vi "Teleop.vi"(10 "Match Info":T1={"Autonomous Elapsed Seconds"=0.0, "TeleOp Elapsed Seconds"=0.0, "Disabled Elapsed Seconds"=0.0, "Visited Autonomous"=FALSE, "Visited TeleOp"=FALSE, "Visited Disabled"=FALSE, "Autonomous Settings"={"Autonomous Style"=enum."Independent", "VI Refnum"=refnum}}, 11 "Call Context":T2) -> ()   [LabVIEW 2012]
doc: "This VI is called for each TeleOp packet received from the DS where the robot is not disabled. It is often used to read from the joysticks and update I/O or to update setpoints for timed control loops. It should complete and return within 20 milliseconds or it may miss DS packets."
uses:
  <vilib>/Rock Robotics/WPI/DriverStation/WPI_DriverStationDerivedRobotMode.ctl
  <vilib>/Rock Robotics/WPI/DriverStation/WPI_DriverStationMatch Info.ctl
  <vilib>/Rock Robotics/WPI/Relay/WPI_RelayValue.ctl
  Robot Global Data.vi
  <vilib>/Rock Robotics/WPI/Joystick/WPI_JoystickGetSetRefNum.vi
panel:
  in  "Hold":dbl=85.0
  in  "Allow Latch":dbl=25.0
  in  "Ext Const":dbl=0.5
  in  "Dep Const":dbl=0.5
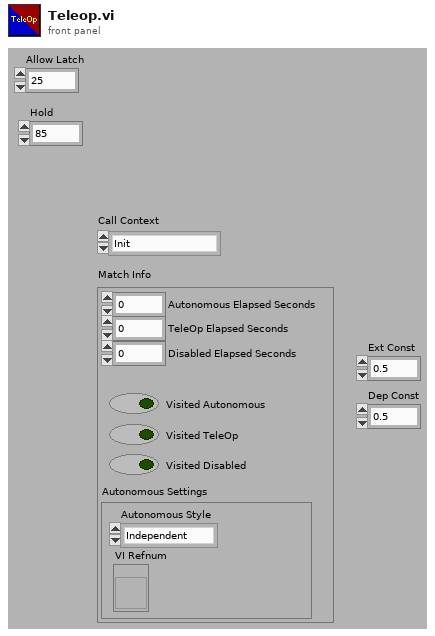
[diagram p1: front panel]
types:
  T1 = typedef "WPI_DriverStationMatch Info.ctl" = cluster{"Autonomous Elapsed Seconds":dbl, "TeleOp Elapsed Seconds":dbl, "Disabled Elapsed Seconds":dbl, "Visited Autonomous":bool, "Visited TeleOp":bool, "Visited Disabled":bool, "Autonomous Settings":cluster{"Autonomous Style":enum16{"Iterative", "Independent"}, "VI Refnum":refnum<vi>}}
  T2 = typedef "WPI_DriverStationDerivedRobotMode.ctl" = enum16{"Init", "Execute", "Stop"}
  T3 = typedef "WPI_RelayValue.ctl" = enum16{"Off", "On", "Forward", "Reverse"}
  T4 = typedef "WPI_ServoDeviceRef.ctl" = cluster{"DeviceStatus":errorcluster, "Digital Module":T5, "PWM Channel":T6, "DeadBand":T7}
  T5 = typedef "FPGA_TypedefDigitalModule.ctl" = enum16{"Digital Module 1", "Digital Module 2"}
  T6 = typedef "FPGA_DIOPWMChannel.ctl" = enum8{"PWM 1", "PWM 2", "PWM 3", "PWM 4", "PWM 5", "PWM 6", "PWM 7", "PWM 8", "PWM 9", "PWM 10", "Invalid"}
  T7 = typedef "WPI_PWMDeadband.ctl" = cluster{"Name":string, "maxPositivePwm":i32, "minPositivePwm":i32, "centerPwm":i32, "maxNegativePwm":i32, "minNegativePwm":i32, "angularRange":u16}
  T8 = typedef "WPI_MotorControlDeviceRef.ctl" = cluster{"DeviceStatus":errorcluster, "Type":enum16{"PWM", "CAN"}, "PWM":cluster{"Digital Module":T5, "PWM Channel":T6, "DeadBand":T7}, "CAN":cluster{"Device Number":u8, "Control Mode":T9, "Semaphore":T10, "Max Vout":dbl}, "Invert":bool, "TransformRef":T11, "InvTransformRef":T11}
  T9 = typedef "WPI_CANJaguar_ControlMode.ctl" = enum8{"Percent VBus", "Current", "Speed", "Position", "Voltage"}
  T10 = typedef "Semaphore RefNum" = refnum<k1>
  T11 = typedef "WPI_PWMTransform_ConPane.ctl" = refnum<vi>
  T12 = cluster{"Driver Station Digital Input (1-8)[0]":bool, "Driver Station Digital Input (1-8)[1]":bool, "Driver Station Digital Input (1-8)[2]":bool, "Driver Station Digital Input (1-8)[3]":bool, "Driver Station Digital Input (1-8)[4]":bool, "Driver Station Digital Input (1-8)[5]":bool, "Driver Station Digital Input (1-8)[6]":bool, "Driver Station Digital Input (1-8)[7]":bool, "Driver Station Digital Input (1-8)[8]":bool}
  T13 = cluster{"Right Servo High":dbl, "Right Servo Mid":dbl, "Right Servo Low":dbl, "Left Servo High":dbl, "Left Servo Mid":dbl, "Left Servo Low":dbl}
  T14 = typedef "WPI_DigitalInputDevRef.ctl" = cluster{"DevStatus":errorcluster, "DIO Channel":T15, "Digital Module":T5}
  T15 = typedef "FPGA_DIOChannel.ctl" = enum8{"DIO 1", "DIO 2", "DIO 3", "DIO 4", "DIO 5", "DIO 6", "DIO 7", "DIO 8", "DIO 9", "DIO 10", "DIO 11", "DIO 12", "DIO 13", "DIO 14", "Invalid"}
  T16 = typedef "WPI_JoystickDevRef.ctl" = cluster{"Device":T17}
  T17 = typedef "WPI_JoystickDeviceEnum.ctl" = enum16{"USB 1", "USB 2", "USB 3", "USB 4", "Kinect 1", "Kinect 2"}
  T18 = cluster{"axis 1 (x)":dbl, "axis 2 (y)":dbl, "axis 3 (throttle)":dbl, "axis 4":dbl, "axis 5":dbl, "axis 6":dbl}
  T19 = typedef "WPI_JoystickButtonState.ctl" = cluster{"Button 1":bool, "Button 2":bool, "Button 3":bool, "Button 4":bool, "Button 5":bool, "Button 6":bool, "Button 7":bool, "Button 8":bool, "Button 9":bool, "Button 10":bool, "Button 11":bool, "Button 12":bool}
  T20 = typedef "WPI_RelayDevRef.ctl" = cluster{"DevStatus":errorcluster, "Relay Channel":T21, "Digital Module":T5, "Relay Direction":T22}
  T21 = typedef "FPGA_DIORelayChannel.ctl" = enum8{"Relay 1", "Relay 2", "Relay 3", "Relay 4", "Relay 5", "Relay 6", "Relay 7", "Relay 8", "Invalid"}
  T22 = typedef "WPI_RelayDirection.ctl" = enum16{"Both directions", "Forward only", "Reverse only"}
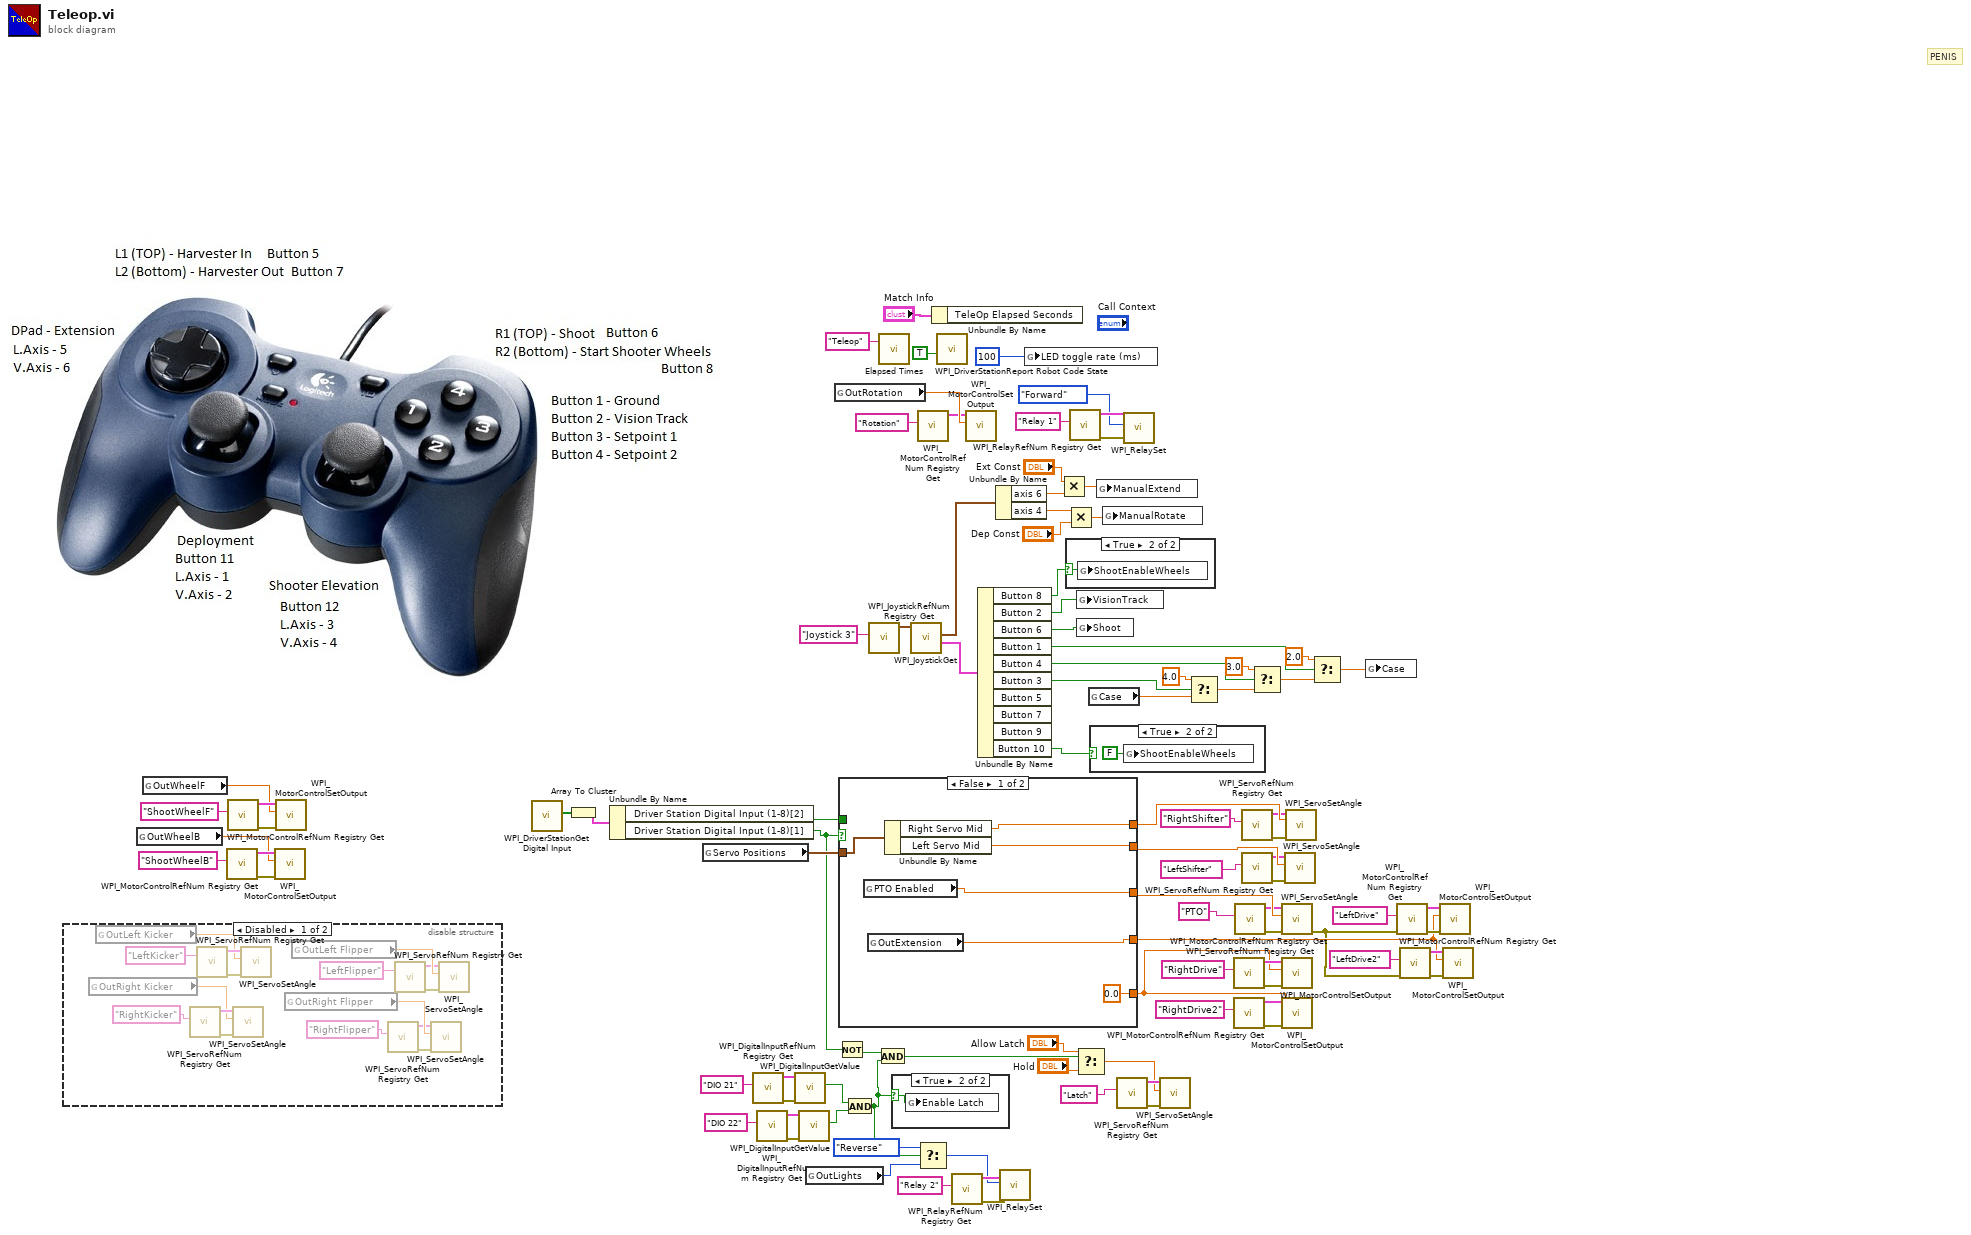
[diagram p0: block diagram]
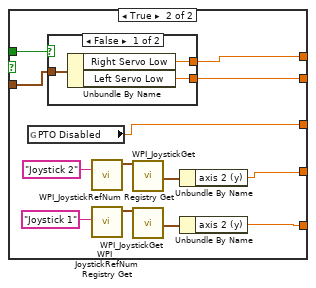
[diagram p4: hidden frame]
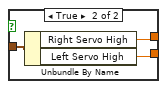
[diagram p5: hidden frame]
diagram:
  # "PENIS"
  n1 = disable-structure shown="Disabled" {
    frame Disabled {
      n2 = global read "Robot Global Data.vi" "OutRight Kicker"() -> (w107:dbl)
      n3 = global read "Robot Global Data.vi" "OutLeft Kicker"() -> (w108:dbl)
      n4 = call <vilib>:"WPI_ServoRefNum Registry Get.vi"("refnum name"="RightKicker") -> ("error out"=w112:errorcluster, "ServoDeviceRef"=w111:T4)  [unwired: 9 in]
      n5 = call <vilib>:"WPI_ServoRefNum Registry Get.vi"("refnum name"="LeftKicker") -> ("error out"=w113:errorcluster, "ServoDeviceRef"=w109:T4)  [unwired: 9 in]
      n6 = call <vilib>:"WPI_ServoSetAngle.vi"("error in (no error)"=w112, "Angle"=w107, "ServoDeviceRef"=w111) -> ()  [unwired: 7 in, 2 out]
      n7 = call <vilib>:"WPI_ServoSetAngle.vi"("error in (no error)"=w113, "Angle"=w108, "ServoDeviceRef"=w109) -> ()  [unwired: 7 in, 2 out]
      n8 = global read "Robot Global Data.vi" "OutRight Flipper"() -> (w106:dbl)
      n9 = global read "Robot Global Data.vi" "OutLeft Flipper"() -> (w105:dbl)
      n10 = call <vilib>:"WPI_ServoRefNum Registry Get.vi"("refnum name"="RightFlipper") -> ("error out"=w101:errorcluster, "ServoDeviceRef"=w102:T4)  [unwired: 9 in]
      n11 = call <vilib>:"WPI_ServoRefNum Registry Get.vi"("refnum name"="LeftFlipper") -> ("error out"=w100:errorcluster, "ServoDeviceRef"=w104:T4)  [unwired: 9 in]
      n12 = call <vilib>:"WPI_ServoSetAngle.vi"("error in (no error)"=w101, "Angle"=w106, "ServoDeviceRef"=w102) -> ()  [unwired: 7 in, 2 out]
      n13 = call <vilib>:"WPI_ServoSetAngle.vi"("error in (no error)"=w100, "Angle"=w105, "ServoDeviceRef"=w104) -> ()  [unwired: 7 in, 2 out]
    }
    frame Enabled {
    }
  }
  n14 = global read "Robot Global Data.vi" "OutWheelB"() -> (w1:dbl)
  n15 = global read "Robot Global Data.vi" "OutWheelF"() -> (w2:dbl)
  n16 = call <vilib>:"WPI_MotorControlRefNum Registry Get.vi"("refnum name"="ShootWheelB") -> ("error out"=w4:errorcluster, "MotorControlDevRef"=w5:T8)  [unwired: 9 in]
  n17 = call <vilib>:"WPI_MotorControlRefNum Registry Get.vi"("refnum name"="ShootWheelF") -> ("error out"=w6:errorcluster, "MotorControlDevRef"=w3:T8)  [unwired: 9 in]
  n18 = call <vilib>:"WPI_MotorControlSetOutput.vi"("error in (no error)"=w4, "Output"=w1, "MotorControlDevRef"=w5) -> ()  [unwired: 6 in, 3 out]
  n19 = call <vilib>:"WPI_MotorControlSetOutput.vi"("error in (no error)"=w6, "Output"=w2, "MotorControlDevRef"=w3) -> ()  [unwired: 6 in, 3 out]
  n20 = call <vilib>:"WPI_DriverStationGet Digital Input.vi"() -> ("Driver Station Digital Input (1-8)"=w64:bool[])  [unwired: 11 in]
  n21 = Array To Cluster(array=w64) -> (cluster=w63:T12)
  n22 = Unbundle By Name(w63) -> ("Driver Station Digital Input (1-8)[2]"=w62:bool, "Driver Station Digital Input (1-8)[1]"=w15:bool)
  n23 = global read "Robot Global Data.vi" "Servo Positions"() -> (w61:T13)
  n24 = call <vilib>:"WPI_DigitalInputRefNum Registry Get.vi"("refnum name"="DIO 21") -> ("error out"=w29:errorcluster, "DigitalInputDevRef"=w22:T14)  [unwired: 9 in]
  n25 = call <vilib>:"WPI_DigitalInputRefNum Registry Get.vi"("refnum name"="DIO 22") -> ("error out"=w26:errorcluster, "DigitalInputDevRef"=w23:T14)  [unwired: 9 in]
  n26 = call <vilib>:"WPI_DigitalInputGetValue.vi"("error in (no error)"=w29, "DigitalInputDevRef"=w22) -> ("Value"=w24:bool)  [unwired: 7 in, 2 out]
  n27 = call <vilib>:"WPI_DigitalInputGetValue.vi"("error in (no error)"=w26, "DigitalInputDevRef"=w23) -> ("Value"=w25:bool)  [unwired: 7 in, 2 out]
  n28 = global read "Robot Global Data.vi" "OutLights"() -> (w21:T3)
  n29 = global read "Robot Global Data.vi" "OutRotation"() -> (w49:dbl)
  n30 = Not(x=w15) -> (.not. x?=w13:bool)
  n31 = case shown="False" w15 {
    tunnel: w62 -> [_ w133]
    tunnel: w61 -> [w120 w132]
    tunnel: [w119 w131] -> w60
    tunnel: [w118 w130] -> w59
    tunnel: [w117 w129] -> w52
    tunnel: [w115 w122] -> w51
    tunnel: [0.0 w121] -> w50
    frame False {
      n32 = global read "Robot Global Data.vi" "PTO Enabled"() -> (w117:dbl)
      n33 = global read "Robot Global Data.vi" "OutExtension"() -> (w115:dbl)
      n34 = Unbundle By Name(w120) -> ("Right Servo Mid"=w119:dbl, "Left Servo Mid"=w118:dbl)
    }
    frame True {
      n35 = global read "Robot Global Data.vi" "PTO Disabled"() -> (w129:dbl)
      n36 = case shown="False" w133 {
        tunnel: w132 -> [w136 w139]
        tunnel: [w135 w138] -> w131
        tunnel: [w134 w137] -> w130
        frame False {
          n37 = Unbundle By Name(w136) -> ("Right Servo Low"=w135:dbl, "Left Servo Low"=w134:dbl)
        }
        frame True {
          n38 = Unbundle By Name(w139) -> ("Right Servo High"=w138:dbl, "Left Servo High"=w137:dbl)
        }
      }
      n39 = call <vilib>:"WPI_JoystickRefNum Registry Get.vi"("refnum name"="Joystick 2") -> ("JoystickDevRef"=w123:T16)  [unwired: 1 in, 9 out]
      n40 = call <vilib>:"WPI_JoystickRefNum Registry Get.vi"("refnum name"="Joystick 1") -> ("JoystickDevRef"=w127:T16)  [unwired: 1 in, 9 out]
      n41 = call <vilib>:"WPI_JoystickGet.vi"("JoystickDevRef"=w123) -> ("Axes"=w125:T18)  [unwired: 1 in, 5 out]
      n42 = call <vilib>:"WPI_JoystickGet.vi"("JoystickDevRef"=w127) -> ("Axes"=w128:T18)  [unwired: 1 in, 5 out]
      n43 = Unbundle By Name(w125) -> ("axis 2 (y)"=w122:dbl)
      n44 = Unbundle By Name(w128) -> ("axis 2 (y)"=w121:dbl)
    }
  }
  n45 = And(x=w24, y=w25) -> (x .and. y?=w14:bool)
  n46 = call <vilib>:"WPI_JoystickRefNum Registry Get.vi"("refnum name"="Joystick 3") -> ("JoystickDevRef"=w95:T16)  [unwired: 9 in, 1 out]
  n47 = And(x=w13, y=w14) -> (x .and. y?=w12:bool)
  n48 = call "Elapsed Times.vi"("Call Name"="Teleop") -> ()  [unwired: 2 in, 1 out]
  n49 = case shown="True" w14 {
    selector: w14 -> [_ w140]
    frame False {
    }
    frame True {
      n50 = global write "Robot Global Data.vi" "Enable Latch"(w140) -> ()
    }
  }
  n51 = call <vilib>:"WPI_JoystickGet.vi"("JoystickDevRef"=w95) -> ("Buttons"=w93:T19, "Axes"=w92:T18)  [unwired: 4 in, 1 out]
  n52 = call <vilib>:"WPI_MotorControlRefNum Registry Get.vi"("refnum name"="Rotation") -> ("MotorControlDevRef"=w47:T8)  [unwired: 9 in, 1 out]
  n53 = Select(t=WPI_RelayValue."Reverse" ("RelayValue"), s=w14, f=w21) -> (s? t:f=w19:T3)
  n54 = Unbundle By Name("Match Info") -> ()  [unwired: 1 out]
  n55 = call <vilib>:"WPI_DriverStationReport Robot Code State.vi"("TeleOp"=TRUE ("Autonomous")) -> ()  [unwired: 10 in, 1 out]
  n56 = call <vilib>:"WPI_RelayRefNum Registry Get.vi"("refnum name"="Relay 2") -> ("error out"=w35:errorcluster, "RelayDevRef"=w33:T20)  [unwired: 9 in]
  n57 = call <vilib>:"WPI_MotorControlSetOutput.vi"("Output"=w49, "MotorControlDevRef"=w47) -> ()  [unwired: 7 in, 3 out]
  n58 = Unbundle By Name(w93) -> ("Button 8"=w79:bool, "Button 2"=w90:bool, "Button 6"=w91:bool, "Button 1"=w89:bool, "Button 4"=w87:bool, "Button 3"=w86:bool, "Button 10"=w78:bool)  [unwired: 3 out]
  n59 = Unbundle By Name(w92) -> ("axis 6"=w32:dbl, "axis 4"=w42:dbl)
  n60 = call <vilib>:"WPI_RelaySet.vi"("error in (no error)"=w35, "RelayValue"=w19, "RelayDevRef"=w33) -> ()  [unwired: 7 in, 2 out]
  n61 = global write "Robot Global Data.vi" "LED toggle rate (ms)"(u32 100 ("LED ms toggle rate")) -> ()
  n62 = Multiply(x="Ext Const", y=w32) -> (x*y=w30:dbl)
  n63 = Multiply(x=w42, y="Dep Const") -> (x*y=w40:dbl)
  n64 = case shown="True" w79 {
    selector: w79 -> [_ w141]
    frame False {
    }
    frame True {
      n65 = global write "Robot Global Data.vi" "ShootEnableWheels"(w141) -> ()
    }
  }
  n66 = call <vilib>:"WPI_RelayRefNum Registry Get.vi"("refnum name"="Relay 1") -> ("error out"=w37:errorcluster, "RelayDevRef"=w39:T20)  [unwired: 9 in]
  n67 = Select(t="Allow Latch", s=w12, f="Hold") -> (s? t:f=w11:dbl)
  n68 = global write "Robot Global Data.vi" "VisionTrack"(w90) -> ()
  n69 = global write "Robot Global Data.vi" "Shoot"(w91) -> ()
  n70 = global read "Robot Global Data.vi" "Case"() -> (w81:dbl)
  n71 = case shown="True" w78 {
    frame False {
    }
    frame True {
      n72 = global write "Robot Global Data.vi" "ShootEnableWheels"(FALSE ("ShootStartWheels")) -> ()
    }
  }
  n73 = global write "Robot Global Data.vi" "ManualExtend"(w30) -> ()
  n74 = global write "Robot Global Data.vi" "ManualRotate"(w40) -> ()
  n75 = call <vilib>:"WPI_ServoRefNum Registry Get.vi"("refnum name"="Latch") -> ("error out"=w18:errorcluster, "ServoDeviceRef"=w16:T4)  [unwired: 9 in]
  n76 = call <vilib>:"WPI_RelaySet.vi"("error in (no error)"=w37, "RelayValue"=WPI_RelayValue."Forward", "RelayDevRef"=w39) -> ()  [unwired: 7 in, 2 out]
  n77 = call <vilib>:"WPI_ServoSetAngle.vi"("error in (no error)"=w18, "Angle"=w11, "ServoDeviceRef"=w16) -> ()  [unwired: 7 in, 2 out]
  n78 = Select(t=4.0, s=w86, f=w81) -> (s? t:f=w85:dbl)
  n79 = call <vilib>:"WPI_MotorControlRefNum Registry Get.vi"("refnum name"="RightDrive") -> ("error out"=w74:errorcluster, "MotorControlDevRef"=w76:T8)  [unwired: 9 in]
  n80 = call <vilib>:"WPI_MotorControlRefNum Registry Get.vi"("refnum name"="RightDrive2") -> ("error out"=w67:errorcluster, "MotorControlDevRef"=w65:T8)  [unwired: 9 in]
  n81 = call <vilib>:"WPI_ServoRefNum Registry Get.vi"("refnum name"="PTO") -> ("error out"=w45:errorcluster, "ServoDeviceRef"=w46:T4)  [unwired: 9 in]
  n82 = call <vilib>:"WPI_ServoRefNum Registry Get.vi"("refnum name"="RightShifter") -> ("error out"=w55:errorcluster, "ServoDeviceRef"=w56:T4)  [unwired: 9 in]
  n83 = call <vilib>:"WPI_ServoRefNum Registry Get.vi"("refnum name"="LeftShifter") -> ("error out"=w57:errorcluster, "ServoDeviceRef"=w58:T4)  [unwired: 9 in]
  n84 = Select(t=3.0, s=w87, f=w85) -> (s? t:f=w83:dbl)
  n85 = call <vilib>:"WPI_ServoSetAngle.vi"("error in (no error)"=w45, "Angle"=w52, "ServoDeviceRef"=w46) -> ("error out"=w41:errorcluster)  [unwired: 7 in, 1 out]
  n86 = call <vilib>:"WPI_MotorControlSetOutput.vi"("error in (no error)"=w74, "Output"=w50, "MotorControlDevRef"=w76) -> ()  [unwired: 6 in, 3 out]
  n87 = call <vilib>:"WPI_MotorControlSetOutput.vi"("error in (no error)"=w67, "Output"=w50, "MotorControlDevRef"=w65) -> ()  [unwired: 6 in, 3 out]
  n88 = call <vilib>:"WPI_ServoSetAngle.vi"("error in (no error)"=w57, "Angle"=w59, "ServoDeviceRef"=w58) -> ()  [unwired: 7 in, 2 out]
  n89 = call <vilib>:"WPI_ServoSetAngle.vi"("error in (no error)"=w55, "Angle"=w60, "ServoDeviceRef"=w56) -> ()  [unwired: 7 in, 2 out]
  n90 = Select(t=2.0, s=w89, f=w83) -> (s? t:f=w80:dbl)
  n91 = global write "Robot Global Data.vi" "Case"(w80) -> ()
  n92 = call <vilib>:"WPI_MotorControlRefNum Registry Get.vi"("error in (no error)"=w41, "refnum name"="LeftDrive") -> ("error out"=w69:errorcluster, "MotorControlDevRef"=w72:T8)  [unwired: 8 in]
  n93 = call <vilib>:"WPI_MotorControlRefNum Registry Get.vi"("error in (no error)"=w41, "refnum name"="LeftDrive2") -> ("error out"=w68:errorcluster, "MotorControlDevRef"=w70:T8)  [unwired: 8 in]
  n94 = call <vilib>:"WPI_MotorControlSetOutput.vi"("error in (no error)"=w69, "Output"=w51, "MotorControlDevRef"=w72) -> ()  [unwired: 6 in, 3 out]
  n95 = call <vilib>:"WPI_MotorControlSetOutput.vi"("error in (no error)"=w68, "Output"=w51, "MotorControlDevRef"=w70) -> ()  [unwired: 6 in, 3 out]
